vi "Create.vi"(9 "Alias":string, 10 "Actor":refnum<class "Actor.lvclass">, 11 "jettl in":refnum<class "jettl.lvclass">) -> (3 "jettl out":refnum<class "jettl.lvclass">)   [LabVIEW 2021, in "jettl.lvlib" / "jettl.lvclass"]
uses:
  jettl.lvclass
  C:/git/jettl/src/Actor/Actor/Actor.lvclass
  Actor/Actor/Actor.lvclass
  State/Nominal State/Nominal State.lvclass
  C:/git/jettl/src/jettl/State/State/State.lvclass
  jettl.lvclass/jettl.ctl
  Actor/Actor/Loop.vi
  jettl.lvlib
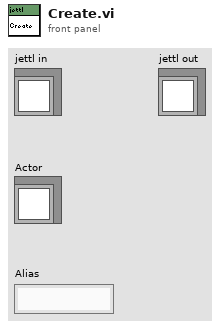
[diagram p1: front panel]
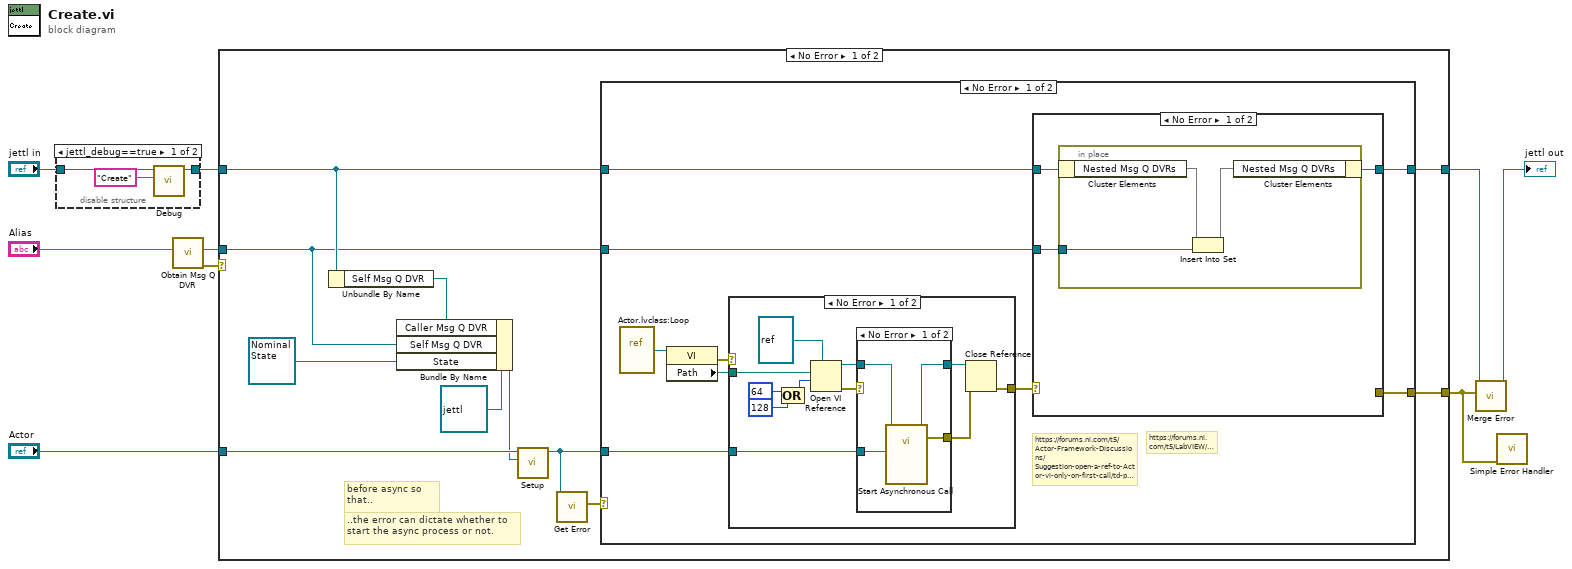
[diagram p0: block diagram]
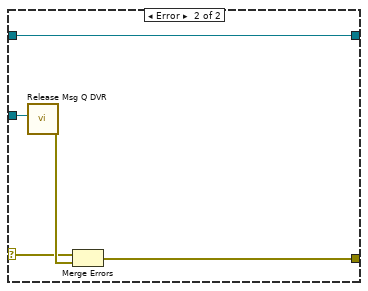
[diagram p5: hidden frame]
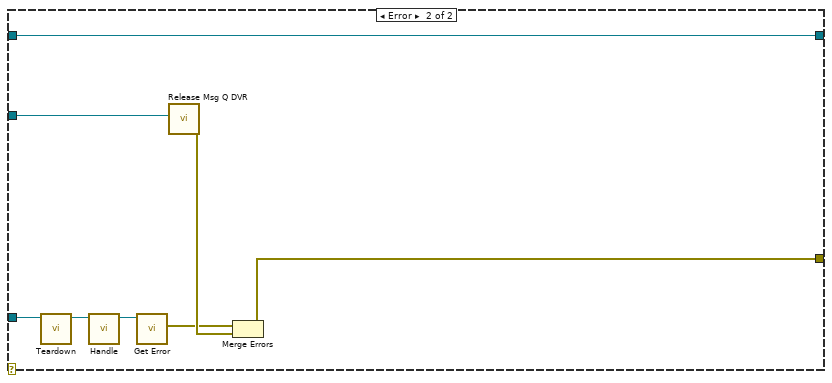
[diagram p6: hidden frame]
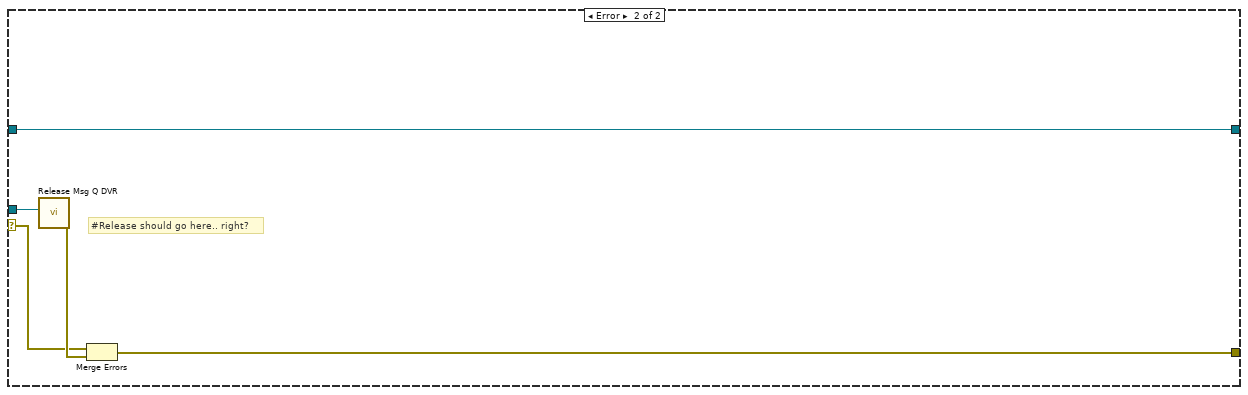
[diagram p7: hidden frame]
diagram:
  n1 = disable-structure shown="jettl_debug==true" {
    disable-tunnel: "jettl in" -> [w12 w13]
    disable-tunnel: [w11 w13] -> w2
    frame condition #0 (active) {
      n2 = call "Debug.vi"("Method"="Create", "jettl in"=w12) -> ("jettl out"=w11:refnum<class "jettl.lvclass">)  [unwired: 9 in]
    }
    frame condition #1 {
    }
  }
  n3 = call "Obtain Msg Q DVR.vi"("Msg Q DVR Alias"="Alias") -> ("error out"=w6:errorcluster, "Msg Q DVR"=w8:refnum<data-value>)  [unwired: 9 in]
  n4 = case shown="No Error" w6 {
    selector: w6 -> [_ w71]
    tunnel: [w24 w75] -> w5
    tunnel: [w23 w73] -> w1
    tunnel: "Actor" -> [w21 _]
    tunnel: w8 -> [w18 w74]
    tunnel: w2 -> [w20 w75]
    frame No Error {
      # "..the error can dictate whether to start the async process or not."
      # "before async so that.."
      n5 = Unbundle By Name(w20) -> ("Self Msg Q DVR"=w19:refnum<data-value>)
      n6 = Bundle By Name(cluster=refnum<class "jettl.lvclass"> refnum ("Self Actor in"), "Caller Msg Q DVR"=w19, "Self Msg Q DVR"=w18, "State"=refnum<class "Nominal State.lvclass"> refnum ("LVCAM.lvlib:Msging Self Actor State.lvclass")) -> (w17:refnum<class "jettl.lvclass">)
      n7 = call-dynamic "Setup.vi"("Actor"=w17, "Actor in"=w21) -> ("Actor out"=w14:refnum<class "Actor.lvclass">)  [unwired: 9 in]
      n8 = call-dynamic "Get Error.vi"("Actor in"=w14) -> ("Error"=w15:errorcluster)  [unwired: 10 in]
      n9 = case shown="No Error" w15 {
        tunnel: [w33 w69] -> w24
        tunnel: w14 -> [w32 w67]
        tunnel: [w31 w68] -> w23
        tunnel: w20 -> [w29 w69]
        tunnel: w18 -> [w28 w70]
        frame No Error {
          # "https://forums.ni.com/t5/LabVIEW/Static-VI-Reference/m-p/3334014#M978333"
          # "https://forums.ni.com/t5/Actor-Framework-Discussions/Suggestion-open-a-ref-to-Actor-vi-only-on-first-call/td-p/3451643/page/4"
          n10 = vi-ref "Actor.lvclass:Loop.vi"() -> (w26:refnum<vi>)
          n11 = property class="VI"(reference=w26) -> (error out=w27:errorcluster, "Path"=w25:path)  [unwired: 1 in, 1 out]
          n12 = case shown="No Error" w27 {
            selector: w27 -> [_ w51]
            tunnel: [w42 w51] -> w30
            tunnel: w25 -> [w38 _]
            tunnel: w32 -> [w34 _]
            frame No Error {
              n13 = Compound Arithmetic op=OR(64 ("options: Multiple Clones,\n  Fire & Forget"), 128 ("options: Multiple Clones,\n  Fire & Forget")) -> (w40:i32)
              n14 = Open VI Reference(type specifier VI Refnum (for type only)=refnum<vi> refnum, vi path=w38, options=w40) -> (vi reference=w36:refnum<vi>, error out=w37:errorcluster)  [unwired: 3 in]
              n15 = case shown="No Error" w37 {
                selector: w37 -> [_ w50]
                tunnel: [w48 w49] -> w44
                tunnel: [w47 w50] -> w43
                tunnel: w36 -> [w46 w49]
                tunnel: w34 -> [w45 _]
                frame No Error {
                  n16 = call-by-ref "Start Asynchronous Call"(reference=w46, "Actor in"=w45) -> (reference out=w48:refnum<vi>, error out=w47:errorcluster)  [unwired: 11 in, 1 out]
                }
                frame Error {
                }
              }
              n17 = Close Reference(reference=w44, error in (no error)=w43) -> (error out=w42:errorcluster)
            }
            frame Error {
            }
          }
          n18 = case shown="No Error" w30 {
            selector: w30 -> [_ w58]
            tunnel: w29 -> [w54 w62]
            tunnel: [w53 w62] -> w33
            tunnel: w28 -> [w52 w61]
            tunnel: [_ w60] -> w31
            frame No Error {
              n19 = in-place {
                in-place-border: w52 -> [w55]
                n20 = in-place-cluster #1(w54) -> ("Nested Msg Q DVRs"=w57:set{refnum<data-value>})
                n21 = Insert Into Set(10:w55, 11:w57) -> (3:w56:set{refnum<data-value>})  [unwired: 1 out]
                n22 = in-place-cluster #1("Nested Msg Q DVRs"=w56) -> (w53:refnum<class "jettl.lvclass">)
              }
            }
            frame Error {
              n23 = call "Release Msg Q DVR.vi"("Msg Q DVR"=w61) -> ("error out"=w59:errorcluster)  [unwired: 10 in]
              n24 = Merge Errors(w58, w59) -> (w60:errorcluster)
            }
          }
        }
        frame Error {
          n25 = call-dynamic "Teardown.vi"("Teardown in"=w67) -> ("Teardown out"=w66:refnum<class "Actor.lvclass">)  [unwired: 10 in]
          n26 = call-dynamic "Handle.vi"("Actor in"=w66) -> ("Actor out"=w65:refnum<class "Actor.lvclass">)  [unwired: 9 in, 1 out]
          n27 = call-dynamic "Get Error.vi"("Actor in"=w65) -> ("Error"=w63:errorcluster)  [unwired: 10 in]
          n28 = call "Release Msg Q DVR.vi"("Msg Q DVR"=w70) -> ("error out"=w64:errorcluster)  [unwired: 10 in]
          n29 = Merge Errors(w63, w64) -> (w68:errorcluster)
        }
      }
    }
    frame Error {
      # "#Release should go here.. right?"
      n30 = call "Release Msg Q DVR.vi"("Msg Q DVR"=w74) -> ("error out"=w72:errorcluster)  [unwired: 10 in]
      n31 = Merge Errors(w71, w72) -> (w73:errorcluster)
    }
  }
  n32 = call-dynamic "Merge Error.vi"("Error"=w1, "jettl in"=w5) -> ("jettl out"=→"jettl out":refnum<class "jettl.lvclass">)  [unwired: 9 in]
  n33 = call <vilib>:"Simple Error Handler.vi"("error in (no error)"=w1) -> ()  [unwired: 4 in, 5 out]
